vi "DAQ Manager.vi"(7 "Enum":T1, 8 "error in":errorcluster, 10 "Sample Rate":i32, 11 "Chl":tag) -> (0 "error out":errorcluster, 2 "data":waveform(dbl)[](array[waveform]))   [LabVIEW 2021]
doc: "This vi has four functions:\nConfig - Creat Channels and set Timer for DAQ, reset Data.\nStart - Start DAQ\nRead - Read DAQ, amd pass out data.\nStop - Clear Channels for DAQ"
uses:
  Control/DAQ Manager Enum.ctl
  <vilib>/DAQmx/read.llb/DAQmx Read (Analog 1D Wfm NChan NSamp).vi
  <vilib>/DAQmx/create/channels.llb/DAQmx Create Channel (AI-Voltage-Basic).vi
  <vilib>/DAQmx/configure/timing.llb/DAQmx Timing (Sample Clock).vi
  <vilib>/DAQmx/miscellaneous.llb/DAQmx Fill In Error Info.vi
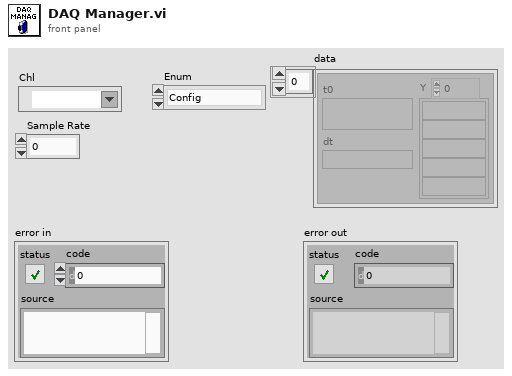
[diagram p1: front panel]
types:
  T1 = typedef "DAQ Manager Enum.ctl" = enum16{"Config", "Start", "Read", "Stop"}
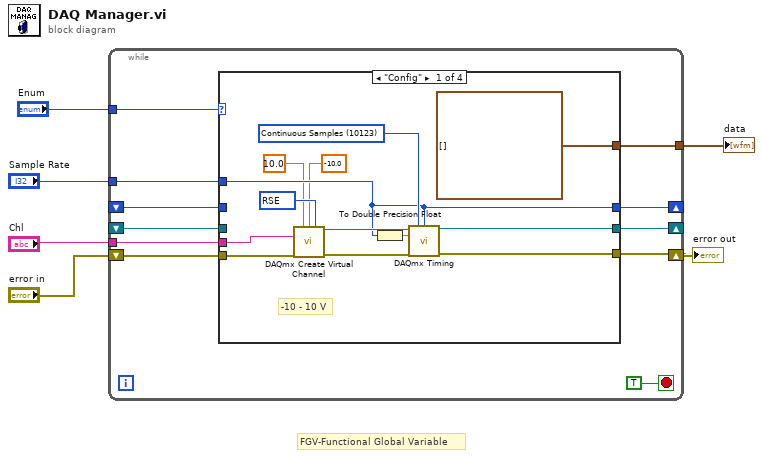
[diagram p0: block diagram]
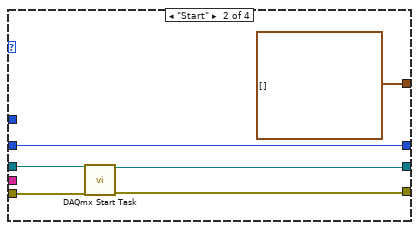
[diagram p2: hidden frame]
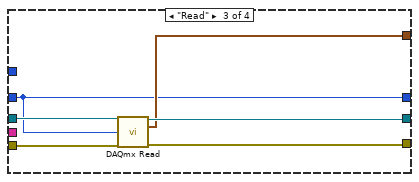
[diagram p3: hidden frame]
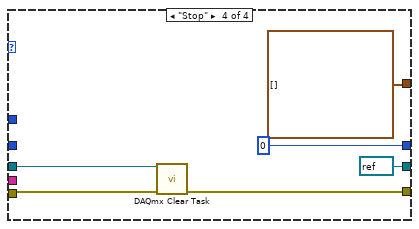
[diagram p4: hidden frame]
diagram:
  # "FGV-Functional Global Variable"
  n1 = while {
    tunnel: "Sample Rate" -> [w17]
    tunnel: "Chl" -> [w16]
    shift-right: [w14] -> _
    shift-left: _ -> [w10]
    shift-right: [w13] -> w3
    shift-left: "error in" -> [w11]
    tunnel: "Enum" -> [w12]
    tunnel: [w9] -> w1
    shift-right: [w8] -> _
    shift-left: _ -> [w7]
    stop <- TRUE stop-if-true
    n2 = case shown="\"Config\"" w12 {
      tunnel: w17 -> [w20 _ _ _]
      tunnel: w16 -> [w25 _ _ _]
      tunnel: [w24 w34 w40 refnum<k21> refnum ("task out")] -> w14
      tunnel: [w23 w33 w39 w46] -> w13
      tunnel: w11 -> [w22 w35 w41 w47]
      tunnel: w10 -> [_ w36 w42 w48]
      tunnel: [waveform(dbl)[] [] ("data") waveform(dbl)[] [] ("data") w38 waveform(dbl)[] [] ("data")] -> w9
      tunnel: [w20 w31 w37 0 ("Sample Rate")] -> w8
      tunnel: w7 -> [_ w31 w37 _]
      frame "Config" {
        w29 = 10123 items=["Finite Samples"=10178, "Continuous Samples"=10123, "Hardware Timed Single Point"=12522] ("sample mode")
        w26 = 10083 items=["Default"=-1, "RSE"=10083, "NRSE"=10078, "Differential"=10106, "Pseudodifferential"=12529] ("input terminal configuration")
        # "-10 - 10 V"
        n3 = call-poly <vilib>:"DAQmx Create Virtual Channel.vi"("maximum value"=10.0, "minimum value"=-10.0, "input terminal configuration"=w26, "physical channels"=w25, "error in"=w22) -> ("task out"=w27:refnum<k21>, "error out"=w28:errorcluster)  [unwired: 9 in]
        n4 = To Double Precision Float(number=w20) -> (double precision float=w30:dbl)
        n5 = call-poly <vilib>:"DAQmx Timing.vi"("task/channels in"=w27, "sample mode"=w29, "samples per channel"=w20, "rate"=w30, "error in"=w28) -> ("task out"=w24:refnum<k21>, "error out"=w23:errorcluster)  [unwired: 9 in]
      }
      frame "Start" {
        n6 = call <vilib>:"DAQmx Start Task.vi"("task/channels in"=w36, "error in"=w35) -> ("task out"=w34:refnum<k21>, "error out"=w33:errorcluster)  [unwired: 12 in]
      }
      frame "Read" {
        n7 = call-poly <vilib>:"DAQmx Read.vi"("task/channels in"=w42, "number of samples per channel"=w37, "error in"=w41) -> ("task out"=w40:refnum<k21>, "data"=w38:waveform(dbl)[], "error out"=w39:errorcluster)  [unwired: 10 in]
      }
      frame "Stop" {
        n8 = call <vilib>:"DAQmx Clear Task.vi"("task in"=w48, "error in"=w47) -> ("error out"=w46:errorcluster)  [unwired: 13 in]
      }
    }
  }
  "error out" <- w3
  "data" <- w1
